vi "Property - Write Allow Home.vi"(4 "error in (no error)":errorcluster, 5 "Value":bool, 6 "Container State":T2, 7 "Display State In":T1={"Header"="", "Label[]"=[], "DisableButtonsLUT"=variant(string[] []), "Menu Config"=variant}) -> (0 "error out":errorcluster, 3 "Display State Out":T1={"Header"="", "Label[]"=[], "DisableButtonsLUT"=variant(string[] []), "Menu Config"=variant})   [LabVIEW 2019, in "Menu Button.xctl"]
doc: "JSMA Module Template - Top Level UI 0.2.0.4\nRob Humfeld - Jet Engineering\nCopyright (c) 2019, Jet Engineering"
uses:
  Menu Button.xctl
  <vilib>/_xctls/Container State.ctl
  State 1.ctl
  <vilib>/_xctls/XControlSupport.lvlib
panel:
  # "Replace the Value Control below with a Control of desired type.\nDo not remove this Control or the others from the connector pane.\nDo not change the connector pane pattern.\nThe Value control should always be the third terminal from top on the input side in the connector pane."
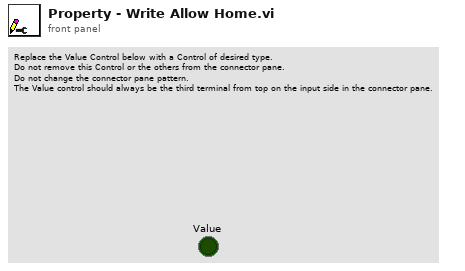
[diagram p1: front panel]
types:
  T1 = typedef "Menu Button.xctl/State 1.ctl" = cluster{"Header":string, "Label[]":string[], "DisableButtonsLUT":variant, "Menu Config":variant}
  T2 = typedef "XControlSupport.lvlib/Container State.ctl" = cluster{"Indicator?":bool, "Run Mode?":bool, " Refnum":refnum<vi>}
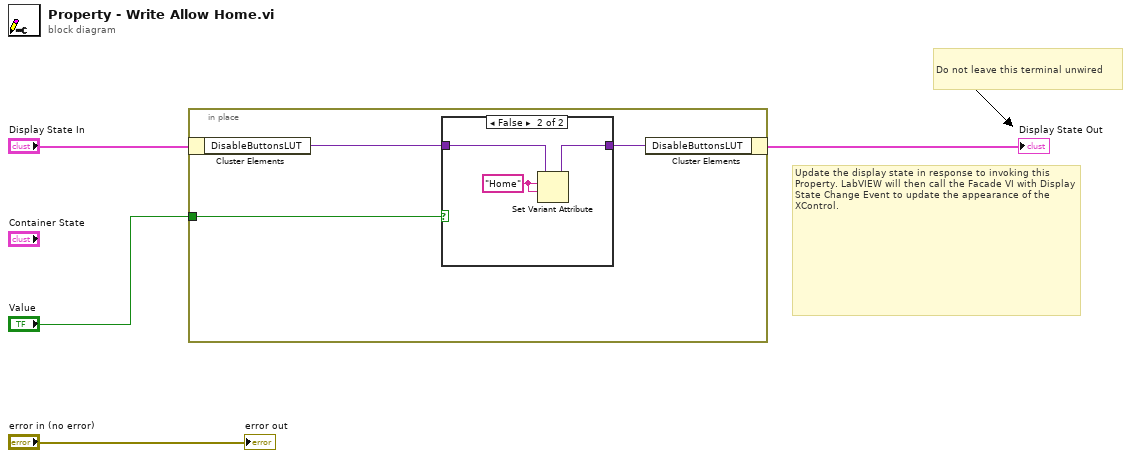
[diagram p0: block diagram]
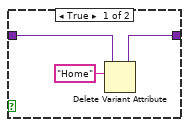
[diagram p2: hidden frame]
diagram:
  # "Do not leave this terminal unwired"
  # "Update the display state in response to invoking this Property. LabVIEW will then call the Facade VI with Display State Change Event to update the appearance of the XControl."
  n1 = in-place {
    in-place-border: "Value" -> [w5]
    n2 = in-place-cluster #1("Display State In") -> ("DisableButtonsLUT"=w6:variant)
    n3 = case shown="False" w5 {
      tunnel: w6 -> [w10 w13]
      tunnel: [w9 w12] -> w7
      frame True {
        n4 = Delete Variant Attribute(6:"Home" ("name"), 7:w10) -> (3:w9:variant)  [unwired: 1 in, 2 out]
      }
      frame False {
        w11 = "Home" ("name")
        n5 = Set Variant Attribute(Variant=w13, name=w11, value=w11) -> (Variant out=w12:variant)  [unwired: 1 in, 2 out]
      }
    }
    n6 = in-place-cluster #1("DisableButtonsLUT"=w7) -> (→"Display State Out":T1)
  }
  "error out" <- "error in (no error)"
